vi "toggleglobal.vi"(6 "toggle input":bool, 7 "set(T)/get(F) tog":bool, 8 "set(T)/get(F) 2":bool, 9 "Thumbinput":bool, 10 "Triggerinput":bool, 11 "set(T)/get(F)":bool) -> (1 "toggleoutput":bool, 2 "Thumboutput":bool, 3 "Boolean 2":bool)   [LabVIEW 2017]
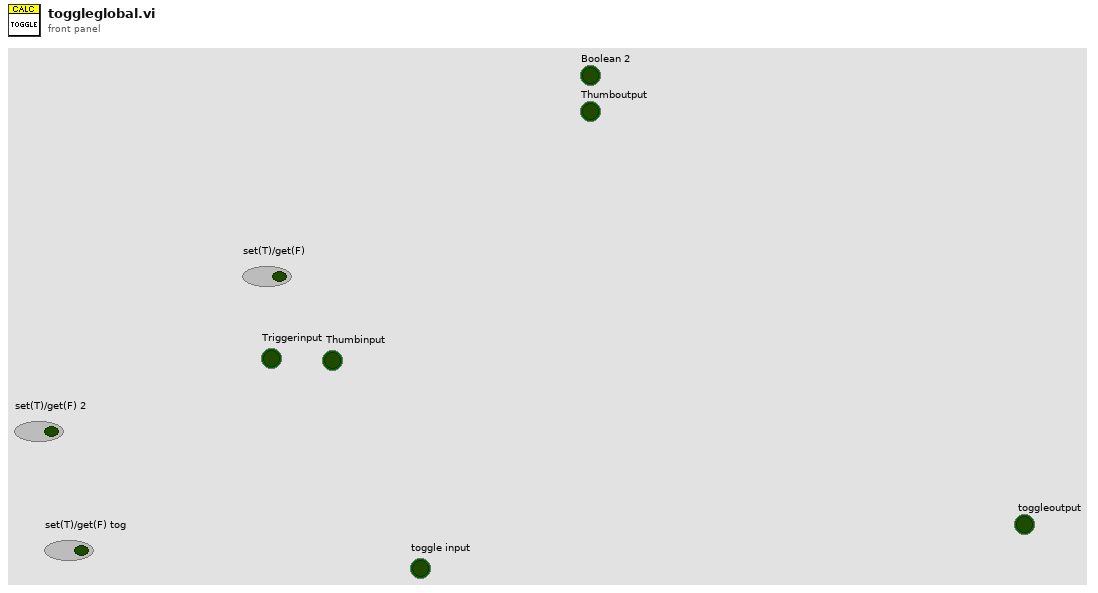
[diagram p1: front panel]
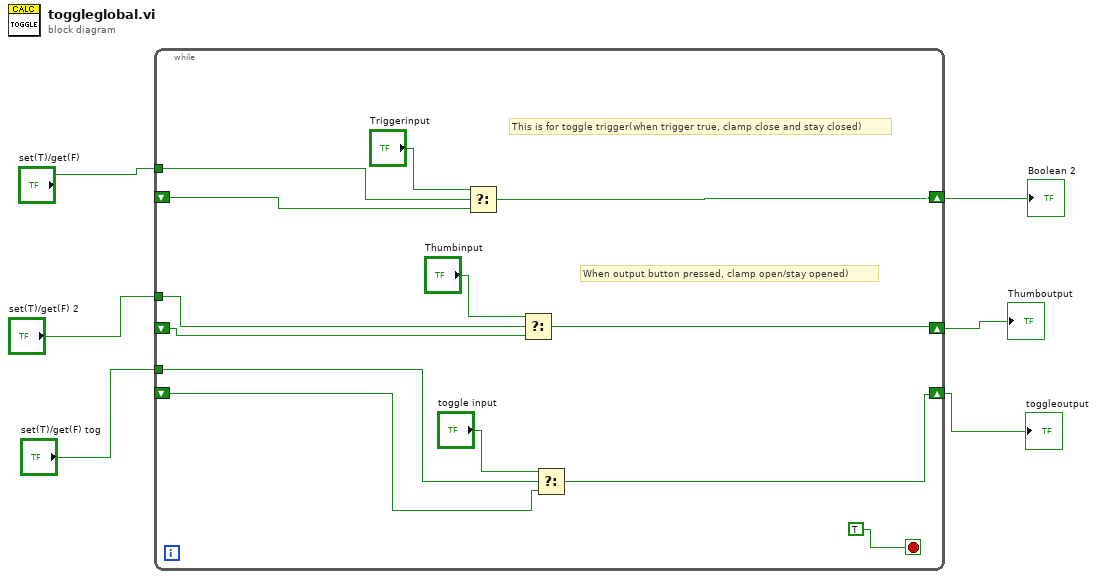
[diagram p0: block diagram]
diagram:
  n1 = while {
    shift-right: [w16] -> w5
    shift-left: _ -> [w19]
    tunnel: "set(T)/get(F)" -> [w18]
    shift-right: [w11] -> w3
    shift-left: _ -> [w13]
    tunnel: "set(T)/get(F) 2" -> [w12]
    shift-right: [w7] -> w1
    shift-left: _ -> [w9]
    tunnel: "set(T)/get(F) tog" -> [w8]
    stop <- TRUE stop-if-true
    # "When output button pressed, clamp open/stay opened)"
    # "This is for toggle trigger(when trigger true, clamp close and stay closed)"
    n2 = Select(t="Triggerinput", s=w18, f=w19) -> (s? t:f=w16:bool)
    n3 = Select(t="Thumbinput", s=w12, f=w13) -> (s? t:f=w11:bool)
    n4 = Select(t="toggle input", s=w8, f=w9) -> (s? t:f=w7:bool)
  }
  "Boolean 2" <- w5
  "Thumboutput" <- w3
  "toggleoutput" <- w1
